vi "Dispatch Transfer Group.vi"(4 "Late Count":i32, 6 "Iteration":u64, 7 "command":T1=enum."Rx", 8 "error in (no error)":errorcluster, 9 "Transfer Group ID":i32, 10 "Plugin ID":i32, 11 "Dispatcher Interface in":refnum<class "Dispatcher Interface.lvclass">) -> (0 "error out":errorcluster, 3 "Dispatcher Interface out":refnum<class "Dispatcher Interface.lvclass">)   [LabVIEW 2017, in "DSF Core.lvlib" / "Dispatcher Interface.lvclass"]
uses:
  Interface/Dispatcher/Dispatcher Interface.lvclass
  Interface/Dispatcher/Command.ctl
  Interface/Dispatcher/Rx Parameters.ctl
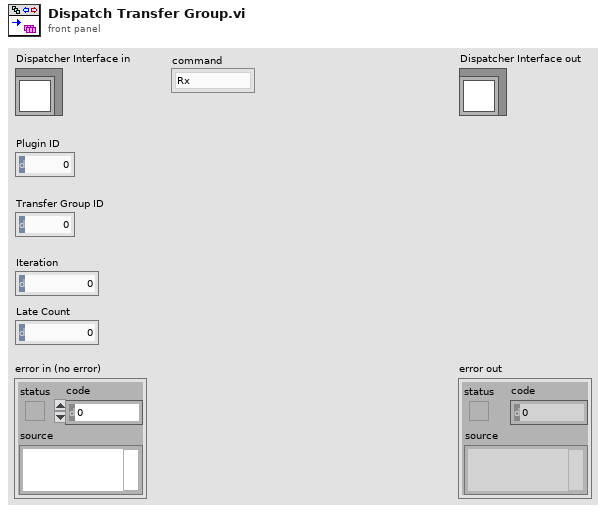
[diagram p1: front panel]
types:
  T1 = typedef "DSF Core.lvlib/Dispatcher Interface.lvclass/Command.ctl" = enum8{"Idle", "Start", "Rx", "Tx", "Set Inline Buffer", "Shutdown", "Error"}
  T2 = typedef "DSF Core.lvlib/Dispatcher Interface.lvclass/Rx Parameters.ctl" = cluster{"Plugin ID":u8, "Transfer Group ID":u8, "unused long":u16, "Late Count":i32, "Iteration":u64}
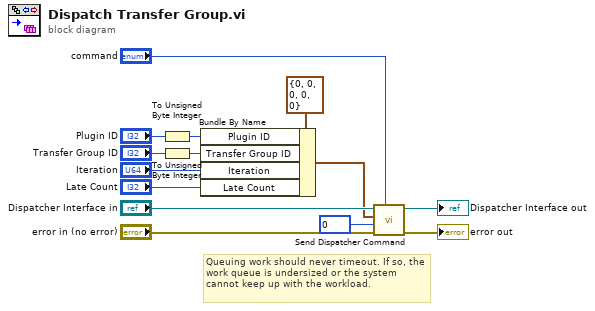
[diagram p0: block diagram]
diagram:
  # "Queuing work should never timeout. If so, the work queue is undersized or the system cannot keep up with the workload."
  n1 = To Unsigned Byte Integer(number="Plugin ID") -> (unsigned 8bit integer=w2:u8)
  n2 = To Unsigned Byte Integer(number="Transfer Group ID") -> (unsigned 8bit integer=w1:u8)
  n3 = Bundle By Name(cluster=T2 {"Plugin ID"=0, "Transfer Group ID"=0, "unused long"=0, "Late Count"=0, "Iteration"=0} ("Rx Parameters"), "Plugin ID"=w2, "Transfer Group ID"=w1, "Iteration"="Iteration", "Late Count"="Late Count") -> (w9:T2)
  n4 = call "Send Dispatcher Command.vi"("Command"="command", "error in (no error)"="error in (no error)", "timeout in ms (0)"=0, "Parameters"=w9, "Dispatcher Interface in"="Dispatcher Interface in") -> ("error out"=→"error out":errorcluster, "Dispatcher Interface out"=→"Dispatcher Interface out":refnum<class "Dispatcher Interface.lvclass">)  [unwired: 5 in]
